vi "Noise Study (FPGA).vi"() -> ()   [LabVIEW 2019]
uses:
  <vilib>/eio/EIONode/EIONode.xnode
  <vilib>/rvi/eio/common/nirviEmuTemplateMethod_errors.vi
  <vilib>/rvi/FXPMathLib/FxpMul/XNode/nifxpmath_Multiplier.xnode
  <vilib>/rvi/FXPMathLib/sim/FxpSim.dll
  <vilib>/Platform/TimedLoop/XDataNode/wakeup.ctl
  <vilib>/Platform/TimedLoop/XDataNode/XDNodeRunTimeDep.lvlib
  <vilib>/Platform/TimedLoop/XDataNode/nitl_modes.ctl
  <vilib>/Platform/TimedLoop/XDataNode/timing_clust.ctl
  <vilib>/Platform/TimedLoop/XDataNode/XDataNode.xnode
  <vilib>/rvi/FXPMathLib/basic elements/FxpIntAccumulator/subVIs/nifxpmath_IntAccumulator_SimConfig.ctl
  <vilib>/rvi/FXPMathLib/basic elements/FxpIntAccumulator/simVIs/DllFxpIntAccumulator_sub.vi
  <vilib>/rvi/FXPMathLib/basic elements/FxpIntAccumulator/XNode/nifxpmath_IntAccumulator.xnode
  <vilib>/fxp/LVFixedPointOverflowPolicyTypeDef.ctl
  <vilib>/rvi/FXPMathLib/FxpSqrt/subVIs/nifxpmath_Sqrt_SimConfig.ctl
  <vilib>/rvi/FXPMathLib/FxpSqrt/simVIs/DllSqrtTemp_sub.vi
  <vilib>/rvi/FXPMathLib/FxpSqrt/XNode/nifxpmath_Sqrt.xnode
  <vilib>/rvi/Analysis/common/codeGenErrors/XNode/niFpgaXNodeCodeGenErrorHandle.vi
  <vilib>/rvi/Analysis/measure/dc-rms/XNode/niFpgaDC-RMS.xnode
  <vilib>/rvi/DataTransferAndStorage/Container/XNode/niFpgaContainer.xnode
  <vilib>/rvi/FXPMathLib/FxpAdd/XNode/nifxpmath_Add.xnode
  <userlib>/_NI SPI IP/FPGA/Controllers/Public/Spi Master Inputs.ctl
  <vilib>/eio/EIOMethodNode/EIOMethodNode.xnode
  Controls/SPI Channels.ctl
  <vilib>/rvi/interface/RandomDataEmulation/nirviRandomDataFpgaReadWriteTemplate.vi
  <vilib>/rvi/Analysis/measure/butterworth/XNode/niFpgaButterworthFilter.xnode
  <vilib>/rvi/FIFO/Fifo_Resource/niFpgaFifoEmulationRefIn.vi
  <userlib>/_NI SPI IP/FPGA/Controllers/Public/Transfer Settings.ctl
panel:
  in  "Filter 2":bool
  in  "index":i32 min=0 max=25 step=1
  in  "Average":bool
  in  "Filter":bool
  out "AI6-31":fxp<+/-,28,17>[](array[numeric])
  in  "DIO63":bool
  in  "AI24-31 Data to Write":u64 format="%.0x"
  out "AI24-31":fxp<+/-,28,17>[](array[numeric])
  out "Read Data 2":u64 format="%.0x"
  in  "AI24-31 Settings":T1 {"Direction Change Bit" max=64 step=1; "Transfer Length (bits)" min=1 max=64 step=1}
  out "AI16-23":fxp<+/-,28,17>[](array[numeric])
  in  "AI16-23 Data to Write":u64 format="%.0x"
  out "Read Data":u64 format="%.0x"
  in  "AI16-23 Settings":T1 {"Direction Change Bit" max=64 step=1; "Transfer Length (bits)" min=1 max=64 step=1}
  in  "AI Divisor":u32
  in  "AO3":fxp<+/-,20,5>
  in  "AO2":fxp<+/-,20,5>
  in  "AO1":fxp<+/-,20,5>
  in  "AO0":fxp<+/-,20,5>
  out "Actual Loop Time":u32
  in  "Loop Timer (uSec)":u32=100
  out "Currents (RMS)":fxp<+/-,28,17>[](array[numeric])
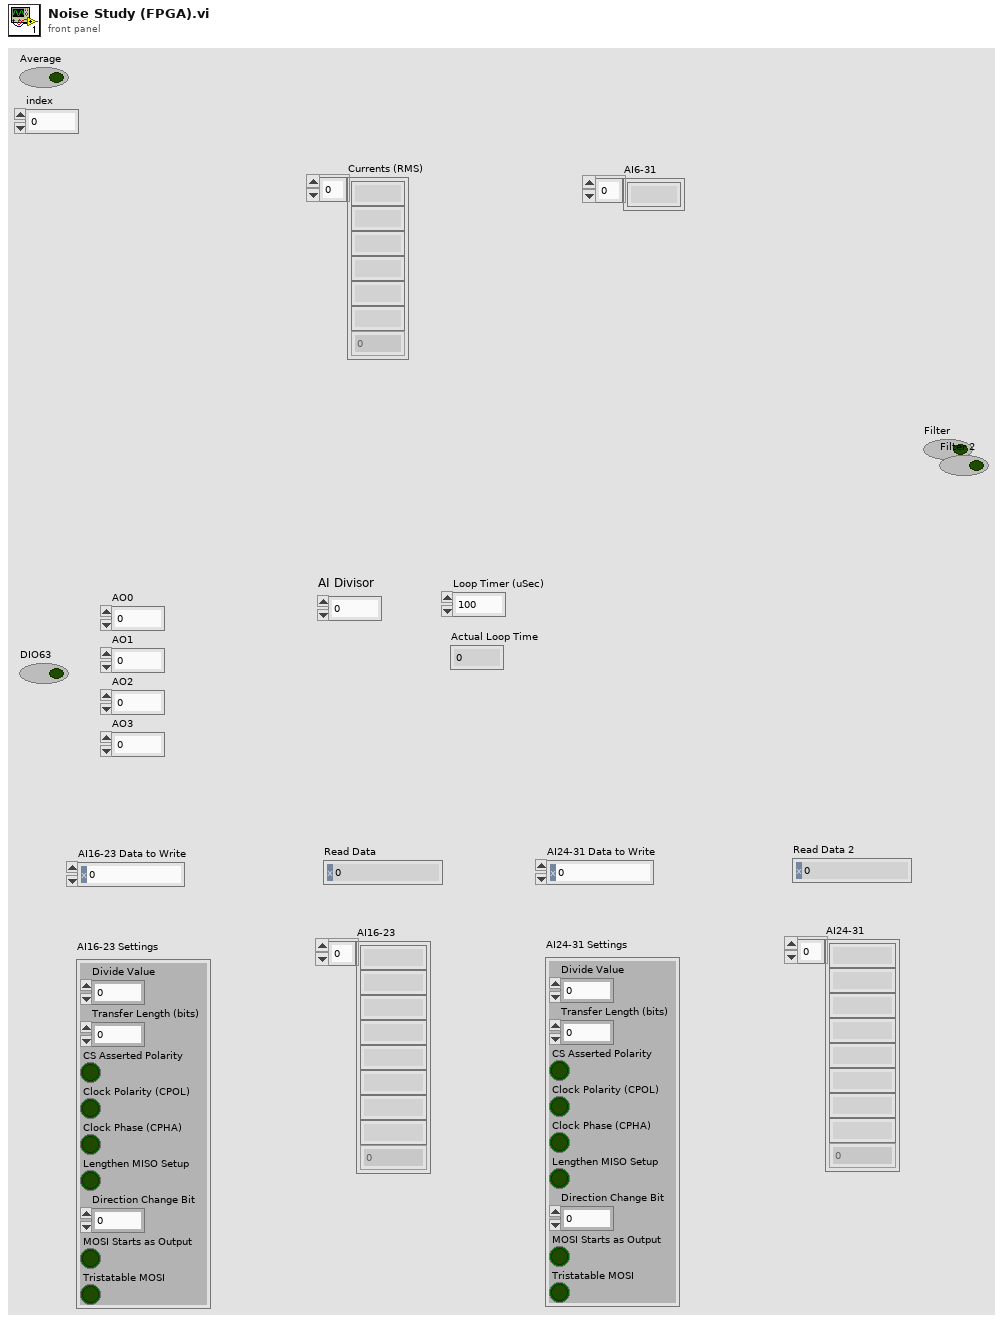
[diagram p1: front panel]
types:
  T1 = typedef "DIO SPI FPGA.lvlib/Transfer Settings.ctl" = cluster{"Divide Value":u8, "Transfer Length (bits)":u8, "CS Asserted Polarity":bool, "Clock Polarity (CPOL)":bool, "Clock Phase (CPHA)":bool, "Lengthen MISO Setup":bool, "Direction Change Bit":u8, "MOSI Starts as Output":bool, "Tristatable MOSI":bool}
  T2 = typedef "SPI Channels.ctl" = cluster{"CS":refnum<k21>, "CLK":refnum<k21>, "MOSI":refnum<k21>, "MISO":refnum<k21>}
  T3 = typedef "XDNodeRunTimeDep.lvlib/timing_clust.ctl" = cluster{"Expected End [f-1]":u64, "Actual End [f-1]":u64, "Finished Late? [f-1]":bool, "Expected End [i-1]":u64, "Actual End [i-1]":u64, "Finished Late? [i-1]":bool, "Expected Start [i]":u64, "Actual Start [i]":u64, "Expected Start [f]":u64, "Actual Start [f]":u64, "Source Name":string, "Structure Name":string, "Period":i64, "Deadline":i64, "Offset":i64, "Start":i64, "Priority":i32, "Timeout":i32, "Mode":T4, "Wakeup Reason":T5, "Error":errorcluster, "Source Type":string, "Secondary Source Type":string, "Global End Time":u64, "Global Start Time":u64, "Frame Duration":u64, "Iteration Duration":u64, "Assigned CPU":i32, "I/O Scan Engine Mode":u32}
  T4 = typedef "XDNodeRunTimeDep.lvlib/nitl_modes.ctl" = enum32{"No Change", "Process missed periods, maintain original phase", "Discard missed periods, maintain original phase", "Process missed periods, ignore original phase", "Discard missed periods, ignore original phase"}
  T5 = typedef "XDNodeRunTimeDep.lvlib/wakeup.ctl" = enum32{"Normal", "Aborted", "Asynchronous wakeup", "Timing source error", "Timed loop error", "Timeout"}
  T6 = typedef "DIO SPI FPGA.lvlib/Spi Master Inputs.ctl" = cluster{"MISO":bool}
  T7 = typedef "DIO SPI FPGA.lvlib/Spi Master Outputs.ctl" = cluster{"Chip Select":bool, "Clock":bool, "MOSI":bool, "MOSI OE":bool}
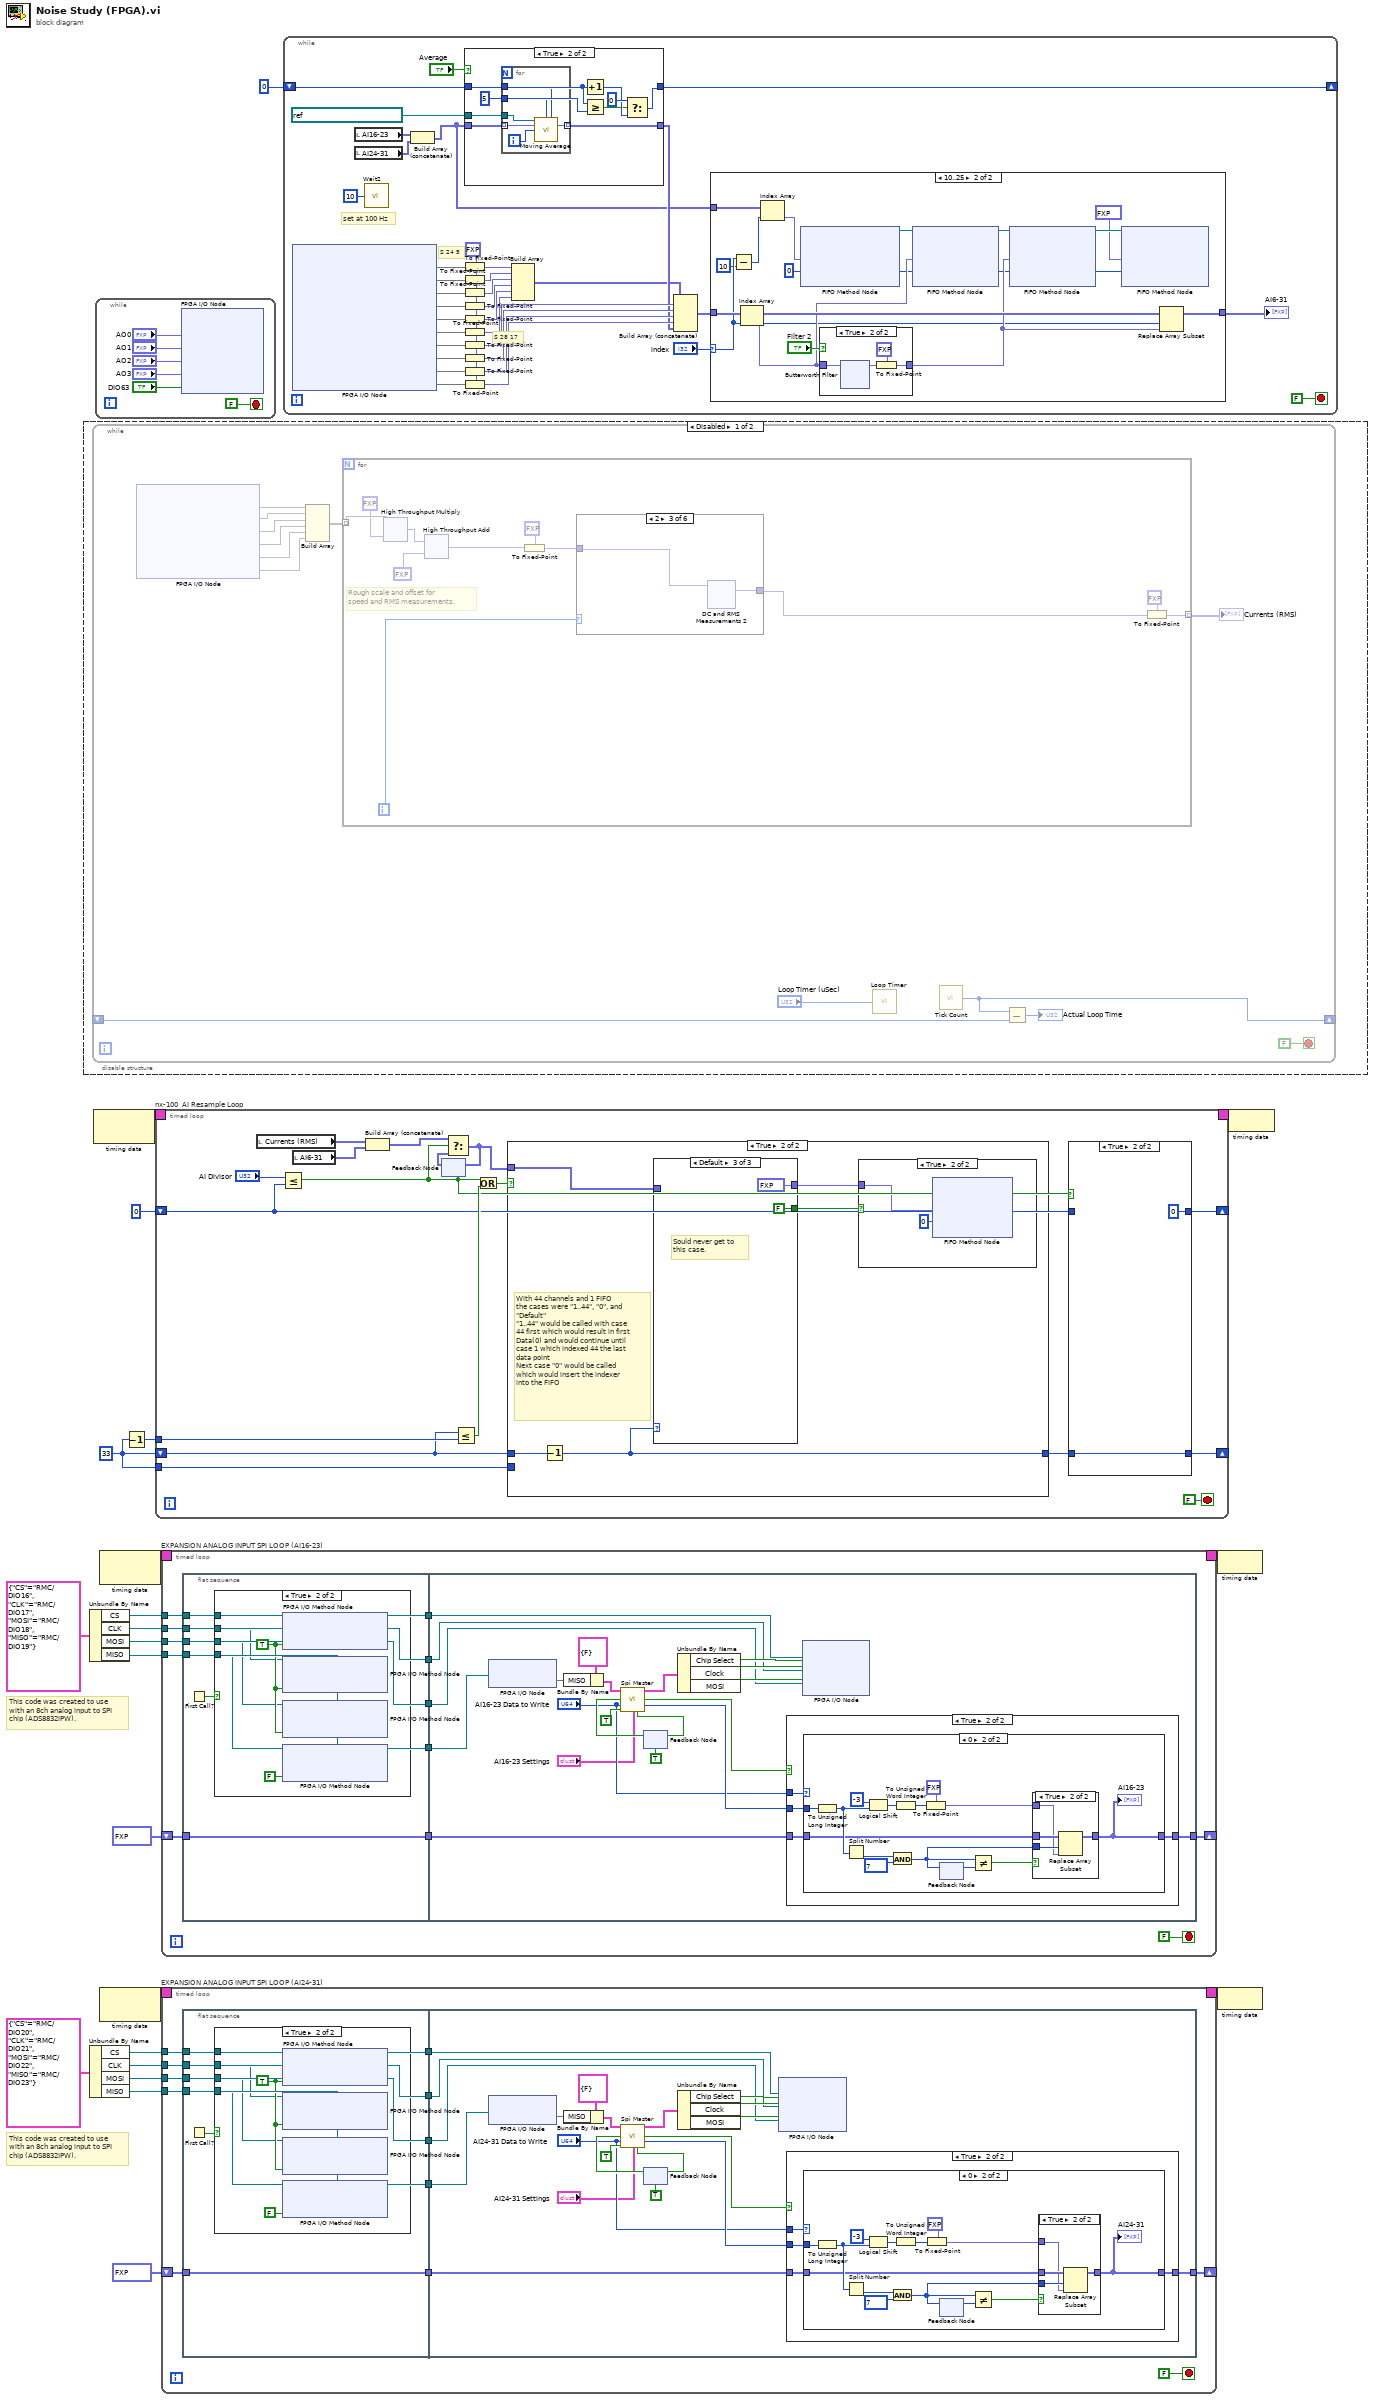
[diagram p0: block diagram]
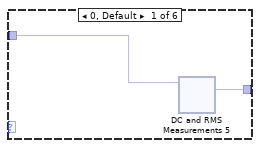
[diagram p2: hidden frame]
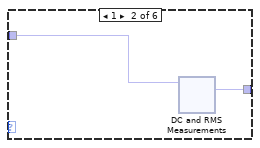
[diagram p3: hidden frame]
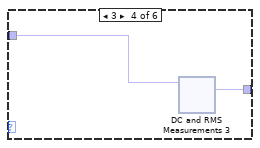
[diagram p4: hidden frame]
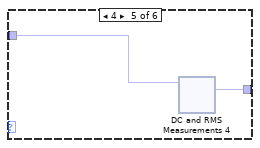
[diagram p5: hidden frame]
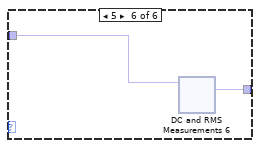
[diagram p6: hidden frame]
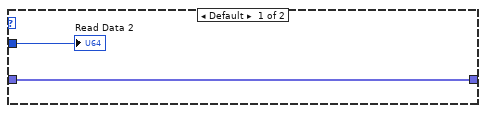
[diagram p10: hidden frame]
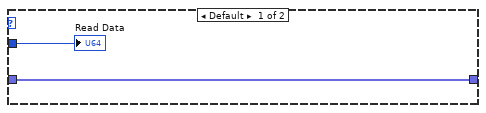
[diagram p14: hidden frame]
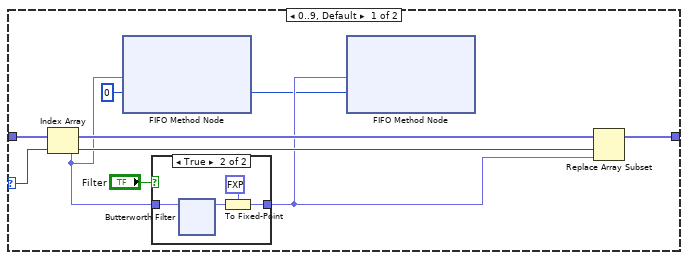
[diagram p16: hidden frame]
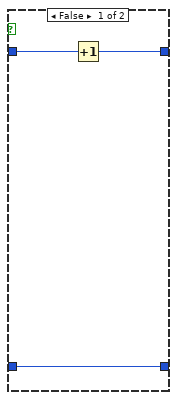
[diagram p20: hidden frame]
diagram:
  w18 = u32 33 ("Sample Divisor")
  # "This code was created to use\nwith an 8ch analog input to SPI\nchip (ADS8832IPW)."
  # "This code was created to use\nwith an 8ch analog input to SPI\nchip (ADS8832IPW)."
  n1 = disable-structure shown="Disabled" {
    frame Disabled {
      n2 = while {
        shift-right: [w26] -> _
        shift-left: _ -> [w25]
        stop <- FALSE stop-if-true
        n3 = xnode "FPGA I/O Node"() -> ("Speed_Current_1 (AI0)"=w29, "Speed_Current_2 (AI1)"=w35, "Speed_Current_3 (AI2)"=w34, "Speed_Current_4 (AI3)"=w33, "Speed_Current_5 (AI4)"=w32, "Speed_Current_6 (AI5)"=w31)  [unwired: 6 in, 6 out]
        n4 = Build Array(w29, w35, w34, w33, w32, w31) -> (w27:void[])
        n5 = for {
          tunnel: w27 -> [w43] mode=indexing
          tunnel: [w36] -> w23 mode=indexing
          i -> [w46]
          # "Rough scale and offset for\nspeed and RMS measurements."
          n6 = xnode ("High Throughput Multiply")("x"=w43, "y"=fxp<+,5,5> 24.0 ("Current Scale")) -> ("x*y"=w44:fxp<+/-,29,10>)
          n7 = xnode ("High Throughput Add")("x"=w44, "y"=fxp<+/-,7,7> -60.0 ("Current Offset")) -> ("x+y"=w39:fxp<+/-,30,11>)
          n8 = To Fixed-Point(fixed-point type=fxp<+/-,26,7> 0.0 ("out"), number=w39) -> (fixed-point=w40:fxp<+/-,26,7>)
          n9 = case shown="2" w46 {
            tunnel: [w48 w158 w268 w378 w488 w598] -> w38
            tunnel: w40 -> [w47 w157 w267 w377 w487 w597]
            frame 0, Default {
              n10 = xnode ("DC and RMS Measurements 5")("input data"=w47) -> ("RMS"=w48:fxp<+,26,7>)  [unwired: 1 in, 1 out]
            }
            frame 1 {
              n11 = xnode ("DC and RMS Measurements")("input data"=w157) -> ("RMS"=w158:fxp<+,26,7>)  [unwired: 1 in, 1 out]
            }
            frame 2 {
              n12 = xnode ("DC and RMS Measurements 2")("input data"=w267) -> ("RMS"=w268:fxp<+,26,7>)  [unwired: 1 in, 1 out]
            }
            frame 3 {
              n13 = xnode ("DC and RMS Measurements 3")("input data"=w377) -> ("RMS"=w378:fxp<+,26,7>)  [unwired: 1 in, 1 out]
            }
            frame 4 {
              n14 = xnode ("DC and RMS Measurements 4")("input data"=w487) -> ("RMS"=w488:fxp<+,26,7>)  [unwired: 1 in, 1 out]
            }
            frame 5 {
              n15 = xnode ("DC and RMS Measurements 6")("input data"=w597) -> ("RMS"=w598:fxp<+,26,7>)  [unwired: 1 in, 1 out]
            }
          }
          n16 = To Fixed-Point(fixed-point type=fxp<+/-,28,17> 0.0 ("out"), number=w38) -> (fixed-point=w36:fxp<+/-,28,17>)
        }
        "Currents (RMS)" <- w23
        n17 = call "Loop Timer"("Count(uSec)"="Loop Timer (uSec)") -> ()  [unwired: 1 out]
        n18 = call "Tick Count"() -> ("Tick Count(uSec)"=w26:u32)
        n19 = Subtract(x=w26, y=w25) -> (x-y=→"Actual Loop Time":u32)
      }
    }
    frame Enabled {
    }
  }
  n20 = Unbundle By Name(T2 {"CS"="RMC/DIO16", "CLK"="RMC/DIO17", "MOSI"="RMC/DIO18", "MISO"="RMC/DIO19"} ("SPI Channels")) -> ("CS"=w10:refnum<k21>, "CLK"=w11:refnum<k21>, "MOSI"=w12:refnum<k21>, "MISO"=w13:refnum<k21>)
  n21 = Unbundle By Name(T2 {"CS"="RMC/DIO20", "CLK"="RMC/DIO21", "MOSI"="RMC/DIO22", "MISO"="RMC/DIO23"} ("SPI Channels")) -> ("CS"=w5:refnum<k21>, "CLK"=w4:refnum<k21>, "MOSI"=w3:refnum<k21>, "MISO"=w2:refnum<k21>)
  n22 = node-c288() -> (w22:T3)  [unwired: 1 in]
  n23 = while {
    stop <- FALSE stop-if-true
    n24 = xnode "FPGA I/O Node"("AO0"="AO0", "AO1"="AO1", "AO2"="AO2", "AO3"="AO3", "RMC/DIO63"="DIO63") -> ()  [unwired: 6 in, 6 out]
  }
  n25 = node-c288() -> (w16:T3)  [unwired: 1 in]
  n26 = node-c288() -> (w8:T3)  [unwired: 1 in]
  n27 = Decrement(x=w18) -> (x-1=w19:u32)
  n28 = timed-loop "nx-100  AI Resample Loop" {
    timing: w22 -> [_]
    timing-out: [_] -> w21
    shift-right: [w728] -> _
    shift-left: u32 0 ("Sample Divisor") -> [w713]
    shift-right: [w727] -> _
    shift-left: w18 -> [w714]
    tunnel: w19 -> [w721]
    tunnel: w18 -> [w720]
    stop <- FALSE stop-if-true
    n29 = local read "Currents (RMS)"() -> (w719:fxp<+/-,28,17>[])
    n30 = Less Or Equal?(x="AI Divisor", y=w713) -> (x <= y?=w717:bool)
    n31 = local read "AI6-31"() -> (w718:fxp<+/-,28,17>[])
    n32 = Build Array (concatenate)(w719, w718) -> (w715:fxp<+/-,28,17>[])
    n33 = feedback #1() -> (w723:fxp<+/-,28,17>[])  [unwired: 1 in]
    n34 = Select(t=w715, s=w717, f=w723) -> (s? t:f=w722:fxp<+/-,28,17>[])
    n35 = feedback-in #1(w722) -> ()
    n36 = Less Or Equal?(x=w714, y=w721) -> (x <= y?=w725:bool)
    n37 = Or(x=w717, y=w725) -> (x .or. y?=w716:bool)
    n38 = case shown="True" w716 {
      tunnel: w714 -> [_ w737]
      tunnel: [w735 w738] -> w724
      tunnel: w722 -> [_ w736]
      tunnel: w720 -> [w735 _]
      frame False {
      }
      frame True {
        # "With 44 channels and 1 FIFO\nthe cases were \"1..44\", \"0\", and\n\"Default\"\n\"1..44\" would be called with case\n44 first which would result in first\nData(0) and would continue until\ncase 1 which indexed 44 the last\ndata point\nNext case \"0\" would be called\nwhich would insert the indexer\ninto the FIFO"
        n39 = Decrement(x=w737) -> (x-1=w738:u32)
        n40 = case shown="Default" w738 {
          selector: w738 -> [w745 _ _]
          tunnel: [w743 fxp<+/-,28,17> -9999.0 ("AI0") fxp<+/-,28,17> -5000.0 ("AI0")] -> w740
          tunnel: [TRUE TRUE FALSE] -> w739
          tunnel: w736 -> [w747 _ _]
          frame 1..32 {
            # "Data case for\nAI Data"
            n41 = Subtract(x=u32 32 ("Sample Divisor"), y=w745) -> (x-y=w744:u32)
            n42 = Index Array(array=w747, index=w744) -> (element=w743:fxp<+/-,28,17>)
          }
          frame 0 {
          }
          frame Default {
            # "Sould never get to\nthis case."
          }
        }
        n43 = case shown="True" w739 {
          tunnel: w740 -> [_ w742]
          frame False {
          }
          frame True {
            n44 = xnode ("FIFO Method Node")("Element"=w742, "Timeout"=0) -> ()  [unwired: 1 in, 2 out]
          }
        }
      }
    }
    n45 = case shown="True" w717 {
      tunnel: w713 -> [w732 _]
      tunnel: [w731 u32 0] -> w728
      tunnel: w724 -> [w730 w733]
      tunnel: [w730 w733] -> w727
      frame False {
        n46 = Increment(x=w732) -> (x+1=w731:u32)
      }
      frame True {
      }
    }
  }
  n47 = timed-loop "EXPANSION ANALOG INPUT SPI LOOP (AI16-23)" {
    timing: w16 -> [_]
    timing-out: [_] -> w15
    shift-right: [w763] -> _
    shift-left: fxp<+/-,28,17>[] [0.0, 0.0, 0.0, 0.0, 0.0, 0.0, 0.0, 0.0] -> [w764]
    tunnel: w10 -> [w762]
    tunnel: w11 -> [w761]
    tunnel: w12 -> [w760]
    tunnel: w13 -> [w759]
    stop <- FALSE stop-if-true
    n48 = flat-sequence {
      tunnel: [w771] -> w765
      tunnel: w764 -> [w771]
      tunnel: w762 -> [w770]
      tunnel: w761 -> [w769]
      tunnel: w760 -> [w768]
      tunnel: w759 -> [w767]
      tunnel: [w770] -> w758
      tunnel: [w769] -> w757
      tunnel: [w768] -> w756
      tunnel: [w767] -> w755
      tunnel: w765 -> [w785]
      tunnel: [w784] -> w763
      tunnel: w758 -> [w783]
      tunnel: w757 -> [w782]
      tunnel: w756 -> [w781]
      tunnel: w755 -> [w780]
      frame #0 {
        n49 = First Call?() -> (First Call?: T/F=w772:bool)
        n50 = case shown="True" w772 {
          tunnel: w770 -> [_ w776]
          tunnel: w769 -> [_ w775]
          tunnel: w768 -> [_ w774]
          tunnel: w767 -> [_ w773]
          frame False {
          }
          frame True {
            w778 = TRUE ("Enable")
            n51 = xnode "FPGA I/O Method Node"("FPGA I/O In"=w776, "Enable"=w778) -> ()  [unwired: 1 out]
            n52 = xnode "FPGA I/O Method Node"("FPGA I/O In"=w775, "Enable"=w778) -> ()  [unwired: 1 out]
            n53 = xnode "FPGA I/O Method Node"("FPGA I/O In"=w774, "Enable"=w778) -> ()  [unwired: 1 out]
            n54 = xnode "FPGA I/O Method Node"("FPGA I/O In"=w773, "Enable"=FALSE) -> ()  [unwired: 1 out]
          }
        }
      }
      frame #1 {
        n55 = xnode "FPGA I/O Node"("FPGA I/O In"=w780) -> ("I/O Item"=w793)  [unwired: 1 out]
        n56 = Bundle By Name(cluster=T6 {"MISO"=FALSE} ("spi input"), "MISO"=w793) -> (w794:T6)
        n57 = feedback #2(TRUE ("read data valid")) -> (w790:bool)
        n58 = call <userlib>:"Spi Master.vi"("spi input"=w794, "start strobe"=w790, "data to write"="AI16-23 Data to Write", "MOSI output enable done"=TRUE, "spi transfer settings"="AI16-23 Settings") -> ("spi output"=w799:T7, "read data valid"=w786:bool, "read data"=w791:u64, "ready for input"=w787:bool)  [unwired: 7 in]
        n59 = feedback-in #2(w787) -> ()
        n60 = Unbundle By Name(w799) -> ("Chip Select"=w798:bool, "Clock"=w797:bool, "MOSI"=w796:bool)
        n61 = case shown="True" w786 {
          tunnel: w791 -> [_ w804]
          tunnel: "AI16-23 Data to Write" -> [_ w803]
          tunnel: w785 -> [w800 w802]
          tunnel: [w800 w801] -> w784
          frame False {
          }
          frame True {
            n62 = case shown="0" w803 {
              tunnel: w804 -> [w806 w820]
              tunnel: w802 -> [w805 w813]
              tunnel: [w805 w812] -> w801
              frame Default {
                "Read Data" <- w806
              }
              frame 0 {
                n63 = To Unsigned Long Integer(number=w820) -> (unsigned 32bit integer=w814:u32)
                n64 = Split Number(x=w814) -> (lo(x)=w818:u16)  [unwired: 1 out]
                n65 = Logical Shift(y=i16 -3, x=w814) -> (x << y=w815:u32)
                n66 = And(x=w818, y=u16 7) -> (x .and. y?=w810:u16)
                n67 = To Unsigned Word Integer(number=w815) -> (unsigned 16bit integer=w807:u16)
                n68 = To Fixed-Point(fixed-point type=fxp<+/-,28,17> 0.0 ("AI0"), number=w807) -> (fixed-point=w808:fxp<+/-,28,17>)
                n69 = feedback #3() -> (w819:u16)  [unwired: 1 in]
                n70 = feedback-in #3(w810) -> ()
                n71 = Not Equal?(x=w810, y=w819) -> (x != y?=w811:bool)
                n72 = case shown="True" w811 {
                  tunnel: w813 -> [w821 w825]
                  tunnel: [w821 w824] -> w812
                  tunnel: w810 -> [_ w823]
                  tunnel: w808 -> [_ w822]
                  frame False {
                  }
                  frame True {
                    n73 = Replace Array Subset(array=w825, new element=w822, index=w823) -> (w824:fxp<+/-,28,17>[])
                  }
                }
                "AI16-23" <- w812
              }
            }
          }
        }
        n74 = xnode "FPGA I/O Node"("I/O Item"=w798, "FPGA I/O In"=w783, "I/O Item"=w797, "FPGA I/O In"=w782, "I/O Item"=w796, "FPGA I/O In"=w781) -> ()  [unwired: 3 out]
      }
    }
  }
  n75 = timed-loop "EXPANSION ANALOG INPUT SPI LOOP (AI24-31)" {
    timing: w8 -> [_]
    timing-out: [_] -> w7
    shift-right: [w836] -> _
    shift-left: fxp<+/-,28,17>[] [0.0, 0.0, 0.0, 0.0, 0.0, 0.0, 0.0, 0.0] -> [w837]
    tunnel: w5 -> [w835]
    tunnel: w4 -> [w834]
    tunnel: w3 -> [w833]
    tunnel: w2 -> [w832]
    stop <- FALSE stop-if-true
    n76 = flat-sequence {
      tunnel: [w844] -> w838
      tunnel: w837 -> [w844]
      tunnel: w835 -> [w843]
      tunnel: w834 -> [w842]
      tunnel: w833 -> [w841]
      tunnel: w832 -> [w840]
      tunnel: [w843] -> w831
      tunnel: [w842] -> w830
      tunnel: [w841] -> w829
      tunnel: [w840] -> w828
      tunnel: w838 -> [w858]
      tunnel: [w857] -> w836
      tunnel: w831 -> [w856]
      tunnel: w830 -> [w855]
      tunnel: w829 -> [w854]
      tunnel: w828 -> [w853]
      frame #0 {
        n77 = First Call?() -> (First Call?: T/F=w845:bool)
        n78 = case shown="True" w845 {
          tunnel: w843 -> [_ w849]
          tunnel: w842 -> [_ w848]
          tunnel: w841 -> [_ w847]
          tunnel: w840 -> [_ w846]
          frame False {
          }
          frame True {
            w851 = TRUE ("Enable")
            n79 = xnode "FPGA I/O Method Node"("FPGA I/O In"=w849, "Enable"=w851) -> ()  [unwired: 1 out]
            n80 = xnode "FPGA I/O Method Node"("FPGA I/O In"=w848, "Enable"=w851) -> ()  [unwired: 1 out]
            n81 = xnode "FPGA I/O Method Node"("FPGA I/O In"=w847, "Enable"=w851) -> ()  [unwired: 1 out]
            n82 = xnode "FPGA I/O Method Node"("FPGA I/O In"=w846, "Enable"=FALSE) -> ()  [unwired: 1 out]
          }
        }
      }
      frame #1 {
        n83 = xnode "FPGA I/O Node"("FPGA I/O In"=w853) -> ("I/O Item"=w866)  [unwired: 1 out]
        n84 = Bundle By Name(cluster=T6 {"MISO"=FALSE} ("spi input"), "MISO"=w866) -> (w867:T6)
        n85 = feedback #4(TRUE ("read data valid")) -> (w863:bool)
        n86 = call <userlib>:"Spi Master.vi"("spi input"=w867, "start strobe"=w863, "data to write"="AI24-31 Data to Write", "MOSI output enable done"=TRUE, "spi transfer settings"="AI24-31 Settings") -> ("spi output"=w872:T7, "read data valid"=w859:bool, "read data"=w864:u64, "ready for input"=w860:bool)  [unwired: 7 in]
        n87 = feedback-in #4(w860) -> ()
        n88 = Unbundle By Name(w872) -> ("Chip Select"=w871:bool, "Clock"=w870:bool, "MOSI"=w869:bool)
        n89 = xnode "FPGA I/O Node"("I/O Item"=w871, "FPGA I/O In"=w856, "I/O Item"=w870, "FPGA I/O In"=w855, "I/O Item"=w869, "FPGA I/O In"=w854) -> ()  [unwired: 3 out]
        n90 = case shown="True" w859 {
          tunnel: w864 -> [_ w877]
          tunnel: "AI24-31 Data to Write" -> [_ w876]
          tunnel: w858 -> [w873 w875]
          tunnel: [w873 w874] -> w857
          frame False {
          }
          frame True {
            n91 = case shown="0" w876 {
              tunnel: w877 -> [w879 w893]
              tunnel: w875 -> [w878 w886]
              tunnel: [w878 w885] -> w874
              frame Default {
                "Read Data 2" <- w879
              }
              frame 0 {
                n92 = To Unsigned Long Integer(number=w893) -> (unsigned 32bit integer=w887:u32)
                n93 = Split Number(x=w887) -> (lo(x)=w891:u16)  [unwired: 1 out]
                n94 = Logical Shift(y=i16 -3, x=w887) -> (x << y=w888:u32)
                n95 = And(x=w891, y=u16 7) -> (x .and. y?=w883:u16)
                n96 = To Unsigned Word Integer(number=w888) -> (unsigned 16bit integer=w881:u16)
                n97 = To Fixed-Point(fixed-point type=fxp<+/-,28,17> 0.0 ("AI0"), number=w881) -> (fixed-point=w880:fxp<+/-,28,17>)
                n98 = feedback #5() -> (w892:u16)  [unwired: 1 in]
                n99 = feedback-in #5(w883) -> ()
                n100 = Not Equal?(x=w883, y=w892) -> (x != y?=w884:bool)
                n101 = case shown="True" w884 {
                  tunnel: w886 -> [w894 w898]
                  tunnel: [w894 w897] -> w885
                  tunnel: w883 -> [_ w896]
                  tunnel: w880 -> [_ w895]
                  frame False {
                  }
                  frame True {
                    n102 = Replace Array Subset(array=w898, new element=w895, index=w896) -> (w897:fxp<+/-,28,17>[])
                  }
                }
                "AI24-31" <- w885
              }
            }
          }
        }
      }
    }
  }
  n103 = while {
    shift-right: [w932] -> _
    shift-left: 0 ("Moving Point Index") -> [w933]
    stop <- FALSE stop-if-true
    w913 = fxp<+/-,28,17> 0.0 ("Controller_Current_1 (AI6)")
    # "S 28 17"
    # "S 24 5"
    # "set at 100 Hz"
    n104 = xnode "FPGA I/O Node"() -> ("Controller_Current_1 (AI6)"=w923, "Controller_Current_2 (AI7)"=w922, "Controller_Current_3 (AI8)"=w921, "Controller_Current_4 (AI9)"=w920, "Controller_Current_5 (AI10)"=w919, "Controller_Current_6 (AI11)"=w918, "Spare_1 (AI12)"=w917, "Temp_1 (AI13)"=w916, "Temp_2 (AI14)"=w915, "PS_Sense (AI15)"=w914)  [unwired: 10 in, 10 out]
    n105 = local read "AI16-23"() -> (w924:fxp<+/-,28,17>[])
    n106 = local read "AI24-31"() -> (w931:fxp<+/-,28,17>[])
    n107 = call "Wait2"("Count(mSec)"=u32 10) -> ()  [unwired: 1 out]
    n108 = Build Array (concatenate)(w924, w931) -> (w901:fxp<+/-,28,17>[])
    n109 = To Fixed-Point(fixed-point type=w913, number=w923) -> (fixed-point=w912:fxp<+/-,28,17>)
    n110 = To Fixed-Point(fixed-point type=w913, number=w922) -> (fixed-point=w911:fxp<+/-,28,17>)
    n111 = To Fixed-Point(fixed-point type=w913, number=w921) -> (fixed-point=w910:fxp<+/-,28,17>)
    n112 = To Fixed-Point(fixed-point type=w913, number=w920) -> (fixed-point=w909:fxp<+/-,28,17>)
    n113 = To Fixed-Point(fixed-point type=w913, number=w919) -> (fixed-point=w908:fxp<+/-,28,17>)
    n114 = To Fixed-Point(fixed-point type=w913, number=w918) -> (fixed-point=w907:fxp<+/-,28,17>)
    n115 = To Fixed-Point(fixed-point type=w913, number=w917) -> (fixed-point=w930:fxp<+/-,28,17>)
    n116 = To Fixed-Point(fixed-point type=w913, number=w916) -> (fixed-point=w929:fxp<+/-,28,17>)
    n117 = To Fixed-Point(fixed-point type=w913, number=w915) -> (fixed-point=w928:fxp<+/-,28,17>)
    n118 = To Fixed-Point(fixed-point type=w913, number=w914) -> (fixed-point=w927:fxp<+/-,28,17>)
    n119 = case shown="True" "Average" {
      tunnel: w933 -> [w987 w993]
      tunnel: [w987 w992] -> w932
      tunnel: w901 -> [w986 w990]
      tunnel: refnum<k21> "Running Avg Memory" ("Memory") -> [_ w989]
      tunnel: [w986 w988] -> w925
      frame False {
      }
      frame True {
        w991 = 5 ("N (# of Ave Pts 8 max)")
        n120 = for {
          tunnel: w993 -> [w997]
          tunnel: w991 -> [w998]
          tunnel: [w1002] -> w988 mode=indexing
          tunnel: w990 -> [w1001] mode=indexing
          tunnel: w989 -> [w1000]
          i -> [w999]
          n121 = call "Moving Average.vi"("Memory In"=w1000, "N (# of Ave Pts 127 max)"=w998, "Moving Point Index"=w997, "Data IN"=w1001, "Channel#"=w999) -> ("Averaged Data"=w1002:fxp<+/-,28,17>)  [unwired: 10 in]
        }
        n122 = Increment(x=w993) -> (x+1=w995:i32)
        n123 = Greater Or Equal?(x=w993, y=w991) -> (x >= y?=w994:bool)
        n124 = Select(t=0, s=w994, f=w995) -> (s? t:f=w992:i32)
      }
    }
    n125 = Build Array(w912, w911, w910, w909, w908, w907) -> (w905:fxp<+/-,28,17>[])
    n126 = Build Array (concatenate)(w905, w930, w929, w928, w927, w925) -> (w904:fxp<+/-,28,17>[])
    n127 = case shown="10..25" "index" {
      selector: "index" -> [w940 w965]
      tunnel: w904 -> [w942 w971]
      tunnel: [w941 w970] -> w902
      tunnel: w901 -> [_ w966]
      frame 0..9, Default {
        w936 = 0 ("Timeout")
        n128 = Index Array(array=w942, index=w940) -> (element=w938:fxp<+/-,28,17>)
        n129 = xnode ("FIFO Method Node")("Element"=w938, "Timeout"=w936) -> ()  [unwired: 1 in, 2 out]
        n130 = case shown="True" "Filter" {
          tunnel: w938 -> [w943 w945]
          tunnel: [w943 w944] -> w937
          frame False {
          }
          frame True {
            n131 = xnode "Butterworth Filter"("input data"=w945) -> ("output data"=w947:fxp<+/-,16,17>)  [unwired: 2 in, 1 out]
            n132 = To Fixed-Point(fixed-point type=fxp<+/-,28,17> 0.0 ("Controller_Current_1 (AI6)"), number=w947) -> (fixed-point=w944:fxp<+/-,28,17>)
          }
        }
        n133 = xnode ("FIFO Method Node")("Element"=w937, "Timeout"=w936) -> ()  [unwired: 1 in, 2 out]
        n134 = Replace Array Subset(array=w942, new element=w937, index=w940) -> (w941:fxp<+/-,28,17>[])
      }
      frame 10..25 {
        w958 = 0 ("Timeout")
        n135 = Subtract(x=w965, y=10) -> (x-y=w963:i32)
        n136 = Index Array(array=w971, index=w965) -> (element=w968:fxp<+/-,28,17>)
        n137 = Index Array(array=w966, index=w963) -> (element=w962:fxp<+/-,28,17>)
        n138 = xnode ("FIFO Method Node")("Element"=w962, "Timeout"=w958) -> ("FIFO Out"=w961:refnum<k21>)  [unwired: 1 in, 1 out]
        n139 = case shown="True" "Filter 2" {
          tunnel: w968 -> [w972 w974]
          tunnel: [w972 w973] -> w967
          frame False {
          }
          frame True {
            n140 = xnode "Butterworth Filter"("input data"=w974) -> ("output data"=w976:fxp<+/-,16,17>)  [unwired: 2 in, 1 out]
            n141 = To Fixed-Point(fixed-point type=fxp<+/-,28,17> 0.0 ("Controller_Current_1 (AI6)"), number=w976) -> (fixed-point=w973:fxp<+/-,28,17>)
          }
        }
        n142 = xnode ("FIFO Method Node")("Element"=w968, "Timeout"=w958, "FIFO In"=w961) -> ("FIFO Out"=w960:refnum<k21>)  [unwired: 1 out]
        n143 = xnode ("FIFO Method Node")("Element"=w967, "Timeout"=w958, "FIFO In"=w960) -> ("FIFO Out"=w959:refnum<k21>)  [unwired: 1 out]
        n144 = xnode ("FIFO Method Node")("Element"=fxp<+/-,28,17> -9999.0, "Timeout"=w958, "FIFO In"=w959) -> ()  [unwired: 2 out]
        n145 = Replace Array Subset(array=w971, new element=w967, index=w965) -> (w970:fxp<+/-,28,17>[])
      }
    }
    "AI6-31" <- w902
  }
  n146 = node-c288(w15) -> ()
  n147 = node-c288(w7) -> ()
  n148 = node-c288(w21) -> ()
